vi "LVClass_DataClient GetHasoSerialNumber.vi"(0 "DataClient in":refnum<class "DataClient.lvclass">, 11 "error in (no error)":errorcluster) -> (4 "DataClient out":refnum<class "DataClient.lvclass">, 8 "Serial":string, 15 "error out":errorcluster)   [LabVIEW 2020, in "DataClient.lvclass"]
doc: "Haso serial number getter.\n\n--------------------------------------------------------------------------------\n\n<B>clientIn </B> : Client object.\n<B>clientOut </B> : Client object.\n<B>serial </B> : Client object.\n<B>ErrorIn </B> : Error\n<B>ErrorOut </B> : Error\n\n--------------------------------------------------------------------------------"
uses:
  DataClient.lvclass
  DataClient.lvclass/DataClient.ctl
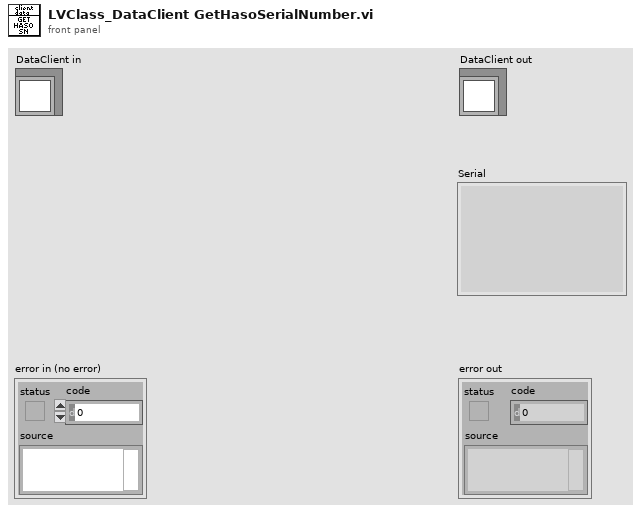
[diagram p1: front panel]
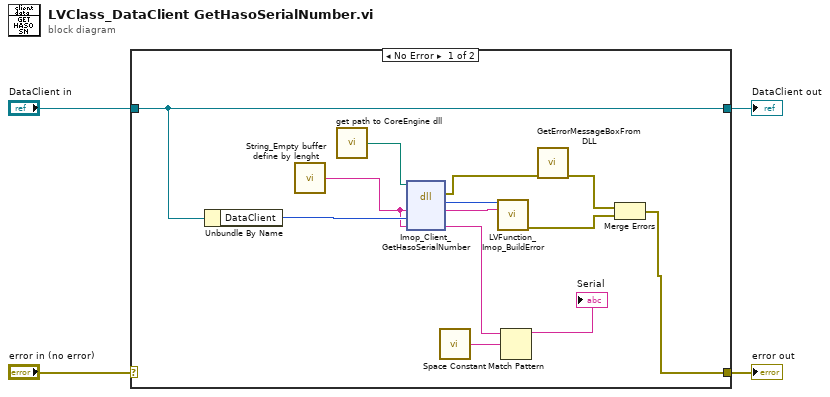
[diagram p0: block diagram]
diagram:
  n1 = case shown="No Error" "error in (no error)" {
    selector: "error in (no error)" -> [_ w19]
    tunnel: [w9 w19] -> w3
    tunnel: [w10 w18] -> w1
    tunnel: "DataClient in" -> [w10 w18]
    frame No Error {
      n2 = Unbundle By Name(w10) -> ("DataClient"=w15:i32)
      n3 = call "String_Empty buffer define by lenght.vi"() -> ("Empty buffer"=w8:string)  [unwired: 1 in]
      n4 = call "get path to CoreEngine dll.vi"() -> ("path to c_interface_vc100.dll"=w13:path)  [unwired: 12 in, 3 out]
      n5 = dll-call lib="D:/soft/HASO_v3/SVN_trunk/ImOpCoreEngine4_LV2011/DLLs/c_interface_vc100.dll" fn="Imop_Client_GetHasoSerialNumber"(path in=w13, "message"=w8, "SlopesServer"=w15, "Serial"=w8) -> (error out=w14:errorcluster, "return type"=w11:i32, "message"=w12:string, "Serial"=w7:string)  [unwired: 3 in, 1 out]
      n6 = call "Space Constant.vi"() -> ("String"=w6:string)
      n7 = call "LVFunction_Imop_BuildError.vi"("code"=w11, "String to Prepend to source (\"\")"=w12) -> ("error out"=w17:errorcluster)  [unwired: 13 in]
      n8 = Match Pattern(string=w7, regular expression=w6) -> (before substring=→"Serial":string)  [unwired: 1 in, 3 out]
      n9 = call "GetErrorMessageBoxFromDLL.vi"("error IN"=w14) -> ("error OUT"=w16:errorcluster)  [unwired: 10 in]
      n10 = Merge Errors(w16, w17) -> (w9:errorcluster)
    }
    frame Error {
    }
  }
  "error out" <- w3
  "DataClient out" <- w1
